vi "Server.vi"() -> ()   [LabVIEW 2021, in "OPC UA.lvlib"]
uses:
  Pfizer Timed Seq/Software/OPC/OPC UA.lvlib
  <vilib>/OPCUA/controls/Supported Security Policies.ctl
  <vilib>/OPCUA/controls/Data Type.ctl
  <vilib>/OPCUA/server/Write Int32.vi
  <vilib>/OPCUA/server/Read Int32.vi
  <vilib>/OPCUA/NI OPC UA Server.lvlib
panel:
  in  "property":T2={"name"="Set Point", "data type"=6, "access level"=3, "description"=""} {"data type" items=["Boolean"=1, "SByte"=2, "Byte"=3, "Int16"=4, "UInt16"=5, "Int32"=6, "UInt32"=7, "Int64"=8, "UInt64"=9, "Float"=10, "Double"=11, "String"=12, "DateTime"=13, "ByteString"=15, "Array of Boolean"=101, "Array of SByte"=102, "Array of Byte"=103, "Array of Int16"=104, "Array of UInt16"=105, "Array of Int32"=106, "Array of UInt32"=107, "Array of Int64"=108, "Array of UInt64"=109, "Array of Float"=110, "Array of Double"=111, "Array of String"=112, "Array of DateTime"=113, "Array of ByteString"=115, "Matrix of Boolean"=201, "Matrix of SByte"=202, "Matrix of Byte"=203, "Matrix of Int16"=204, "Matrix of UInt16"=205, "Matrix of Int32"=206, "Matrix of UInt32"=207, "Matrix of Int64"=208, "Matrix of UInt64"=209, "Matrix of Float"=210, "Matrix of Double"=211, "Matrix of String "=212, "Matrix of DateTime"=213, "Matrix of ByteString"=215]; "access level" items=["read-only"=1, "write-only"=2, "read/write"=3]}
  in  "item":T2={"name"="Node", "data type"=6, "access level"=3, "description"=""} {"data type" items=["Boolean"=1, "SByte"=2, "Byte"=3, "Int16"=4, "UInt16"=5, "Int32"=6, "UInt32"=7, "Int64"=8, "UInt64"=9, "Float"=10, "Double"=11, "String"=12, "DateTime"=13, "ByteString"=15, "Array of Boolean"=101, "Array of SByte"=102, "Array of Byte"=103, "Array of Int16"=104, "Array of UInt16"=105, "Array of Int32"=106, "Array of UInt32"=107, "Array of Int64"=108, "Array of UInt64"=109, "Array of Float"=110, "Array of Double"=111, "Array of String"=112, "Array of DateTime"=113, "Array of ByteString"=115, "Matrix of Boolean"=201, "Matrix of SByte"=202, "Matrix of Byte"=203, "Matrix of Int16"=204, "Matrix of UInt16"=205, "Matrix of Int32"=206, "Matrix of UInt32"=207, "Matrix of Int64"=208, "Matrix of UInt64"=209, "Matrix of Float"=210, "Matrix of Double"=211, "Matrix of String "=212, "Matrix of DateTime"=213, "Matrix of ByteString"=215]; "access level" items=["read-only"=1, "write-only"=2, "read/write"=3]}
  in  "supported security policies (None)":T3={"None"=TRUE, "Sign with Basic128Rsa15"=TRUE, "Sign and Encrypt with Basic128Rsa15"=TRUE, "Sign with Basic256"=TRUE, "Sign and Encrypt with Basic256"=TRUE}
  out "server endpoint URL":string
  in  "stop":bool
  out "Device.Node":i32
  out "Device.Node.Set Point":i32
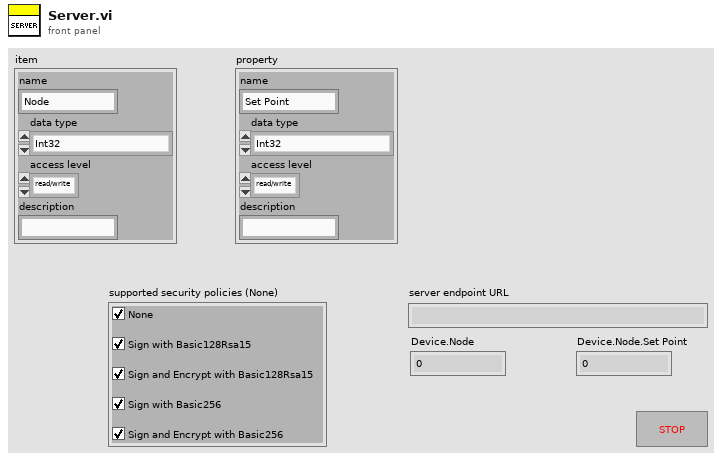
[diagram p1: front panel]
types:
  T1 = typedef "Data Type.ctl" = u16
  T2 = cluster{"name":string, "data type":T1, "access level":u16, "description":string}
  T3 = typedef "Supported Security Policies.ctl" = cluster{"None":bool, "Sign with Basic128Rsa15":bool, "Sign and Encrypt with Basic128Rsa15":bool, "Sign with Basic256":bool, "Sign and Encrypt with Basic256":bool}
  T4 = typedef "OPC UA Server Refnum.ctl" = refnum<k21>
  T5 = typedef "NodeId.ctl" = string
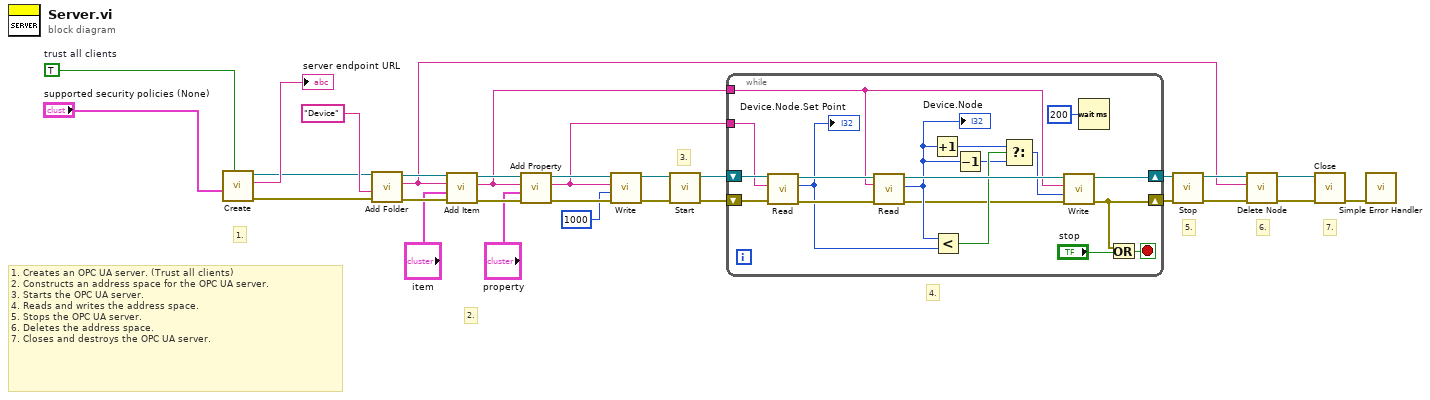
[diagram p0: block diagram]
diagram:
  w1 = TRUE  # trust all clients
  # "1. Creates an OPC UA server. (Trust all clients)\n2. Constructs an address space for the OPC UA server.\n3. Starts the OPC UA server.\n4. Reads and writes the address space.\n5. Stops the OPC UA server.\n6. Deletes the address space.\n7. Closes and destroys the OPC UA server."
  # "7."
  # "6."
  # "5."
  # "4."
  # "3."
  # "2."
  # "1."
  n1 = call <vilib>:"Create.vi"("trust all clients (F)"=w1, "supported security policies (None)"="supported security policies (None)") -> ("error out"=w2:errorcluster, "server endpoint URL"=→"server endpoint URL":string, "OPC UA server refnum out"=w3:T4)  [unwired: 7 in]
  n2 = call <vilib>:"Add Folder.vi"("error in (no error)"=w2, "folder name"="Device", "OPC UA server refnum in"=w3) -> ("error out"=w28:errorcluster, "folder node ID"=w16:T5, "OPC UA server refnum out"=w29:T4)  [unwired: 5 in]
  n3 = call <vilib>:"Add Item.vi"("error in (no error)"=w28, "item"="item", "parent folder node ID"=w16, "OPC UA server refnum in"=w29) -> ("error out"=w18:errorcluster, "item node ID"=w12:T5, "OPC UA server refnum out"=w27:T4)  [unwired: 3 in, 1 out]
  n4 = call <vilib>:"Add Property.vi"("error in (no error)"=w18, "property"="property", "item node ID"=w12, "OPC UA server refnum in"=w27) -> ("error out"=w17:errorcluster, "property node ID"=w8:T5, "OPC UA server refnum out"=w19:T4)  [unwired: 3 in, 1 out]
  n5 = call-poly <vilib>:"Write.vi"("error in (no error)"=w17, "value"=1000, "node ID"=w8, "OPC UA server refnum in"=w19) -> ("error out"=w7:errorcluster, "OPC UA server refnum out"=w6:T4)  [unwired: 5 in, 1 out]
  n6 = call <vilib>:"Start.vi"("error in (no error)"=w7, "OPC UA server refnum in"=w6) -> ("error out"=w4:errorcluster, "OPC UA server refnum out"=w5:T4)  [unwired: 7 in, 1 out]
  n7 = while {
    tunnel: w12 -> [w40]
    shift-right: [w45] -> w23
    shift-left: w5 -> [w44]
    shift-right: [w31] -> w21
    shift-left: w4 -> [w47]
    tunnel: w8 -> [w43]
    stop <- w32 stop-if-true
    n8 = call-poly <vilib>:"Read.vi"("error in (no error)"=w47, "node ID"=w43, "OPC UA server refnum in"=w44) -> ("error out"=w41:errorcluster, "value"=w39:i32, "OPC UA server refnum out"=w48:T4)  [unwired: 4 in, 2 out]
    "Device.Node.Set Point" <- w39
    n9 = call-poly <vilib>:"Read.vi"("error in (no error)"=w41, "node ID"=w40, "OPC UA server refnum in"=w48) -> ("error out"=w33:errorcluster, "value"=w35:i32, "OPC UA server refnum out"=w42:T4)  [unwired: 4 in, 2 out]
    "Device.Node" <- w35
    n10 = Increment(x=w35) -> (x+1=w37:i32)
    n11 = Less?(x=w35, y=w39) -> (x < y?=w38:bool)
    n12 = Decrement(x=w35) -> (x-1=w36:i32)
    n13 = Select(t=w37, s=w38, f=w36) -> (s? t:f=w34:i32)
    n14 = call-poly <vilib>:"Write.vi"("error in (no error)"=w33, "value"=w34, "node ID"=w40, "OPC UA server refnum in"=w42) -> ("error out"=w31:errorcluster, "OPC UA server refnum out"=w45:T4)  [unwired: 5 in, 1 out]
    n15 = Wait (ms)(milliseconds to wait=u32 200) -> ()  [unwired: 1 out]
    n16 = Or(x=w31, y="stop") -> (x .or. y?=w32:bool)
  }
  n17 = call <vilib>:"Stop.vi"("error in (no error)"=w21, "OPC UA server refnum in"=w23) -> ("error out"=w20:errorcluster, "OPC UA server refnum out"=w22:T4)  [unwired: 8 in]
  n18 = call <vilib>:"Delete Node.vi"("error in (no error)"=w20, "node ID"=w16, "OPC UA server refnum in"=w22) -> ("error out"=w24:errorcluster, "OPC UA server refnum out"=w25:T4)  [unwired: 7 in]
  n19 = call <vilib>:"Close.vi"("error in (no error)"=w24, "OPC UA server refnum in"=w25) -> ("error out"=w11:errorcluster)  [unwired: 9 in]
  n20 = call <vilib>:"Simple Error Handler.vi"("error in (no error)"=w11) -> ()  [unwired: 4 in, 5 out]
